vi "Calculate Splitter Height.vi"(8 "error in (no error)":errorcluster, 10 "Panel Bounds":T1, 11 "Splitter Height":i32) -> (0 "error out":errorcluster, 3 "Splitter Height":i32)   [LabVIEW 2015, in "ScriptDialog.lvclass"]
uses:
  ScriptDialog.lvclass
  <vilib>/Utility/miscctls.llb/LVBoundsTypeDef.ctl
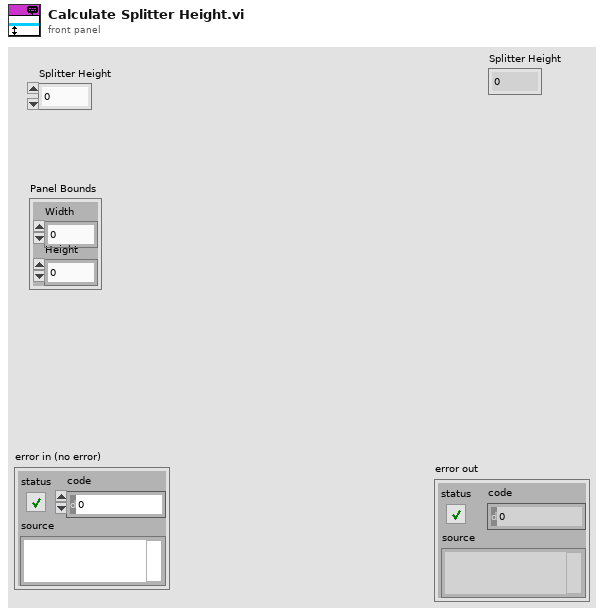
[diagram p1: front panel]
types:
  T1 = typedef "LVBoundsTypeDef.ctl" = cluster{"Width":u32, "Height":u32}
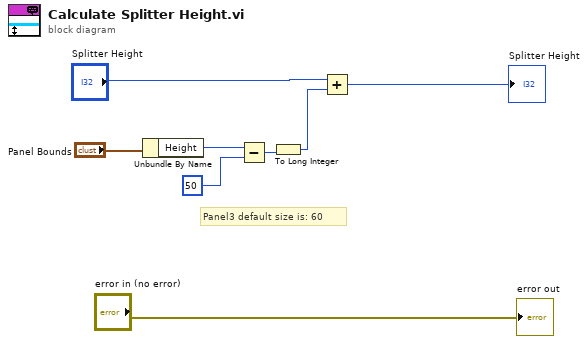
[diagram p0: block diagram]
diagram:
  # "Panel3 default size is: 60"
  n1 = Unbundle By Name("Panel Bounds") -> ("Height"=w7:u32)
  n2 = Subtract(x=w7, y=u32 50) -> (x-y=w5:u32)
  n3 = To Long Integer(number=w5) -> (32bit integer=w4:i32)
  n4 = Add(x="Splitter Height", y=w4) -> (x+y=→"Splitter Height":i32)
  "error out" <- "error in (no error)"
